vi "Read Has errors.vi"(11 "CDependencyInspection in":refnum<class "CDependencyInspection.lvclass">) -> (1 "empty?":bool, 3 "CDependencyInspection out":refnum<class "CDependencyInspection.lvclass">)   [LabVIEW 2020, in "DependencyInspection.lvlib" / "CDependencyInspection.lvclass"]
uses:
  CDependencyInspection.lvclass
  ErrorManager/ErrorManager/ErrorManager.lvclass
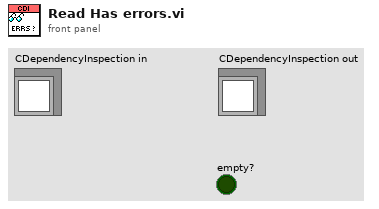
[diagram p1: front panel]
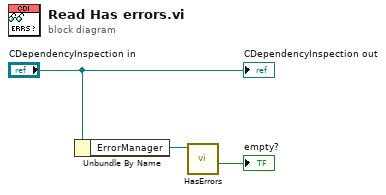
[diagram p0: block diagram]
diagram:
  n1 = Unbundle By Name("CDependencyInspection in") -> ("ErrorManager"=w2:refnum<class "ErrorManager.lvclass">)
  n2 = call-dynamic "HasErrors.vi"("ErrorManager in"=w2) -> ("empty?"=→"empty?":bool)  [unwired: 8 in, 2 out]
  "CDependencyInspection out" <- "CDependencyInspection in"
